vi "Event Log.Show.vi"(8 "error in":errorcluster) -> (0 "error out":errorcluster)   [LabVIEW 2024, in "EQMF.lvlib" / "Event Log.lvlib"]
uses:
  Event Log.lvlib
  Module/Window/Window.Task, Action.ctl
  Module/Module Utils.lvlib
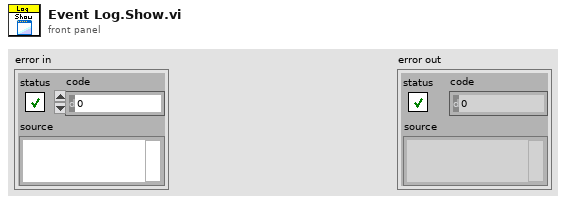
[diagram p1: front panel]
types:
  T1 = typedef "EQMF.lvlib/Module Utils.lvlib/Window.Task, Action.ctl" = enum16{"Resize()", "Show Panel(Bool)", "Show Scroll Bars(Bool)", "Dock to SubPanel(SubPanel Ref)", "Undock from SubPanel()", "Return to SubPanel()", "Go To Maint Tab()", "Show Maint Tab(Bool)", "Open Block Diagram()"}
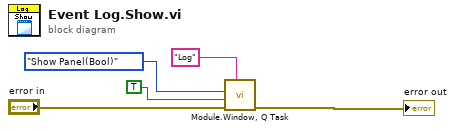
[diagram p0: block diagram]
diagram:
  n1 = call "Module.Window, Q Task.vi"("Q Name"="Log" ("name (unnamed)"), "error in"="error in", "Show"=TRUE, "Action"=Window.Task,_Action."Show Panel(Bool)") -> ("error out"=→"error out":errorcluster)  [unwired: 6 in, 1 out]
